vi "my_4th_vi_noloop.vi"(9 "error in (no error)":errorcluster, 10 "Color range":T2, 11 "PNG file":path) -> (2 "error out":errorcluster, 3 "Billard rect":T1)   [LabVIEW 2019]
uses:
  <vilib>/Analysis/Matrix/Numeric/Conversions/Array To Matrix - RA2.vi
  <vilib>/Analysis/Matrix/Numeric/Multiply/Multiply - RM,RM.vi
  <vilib>/Analysis/Matrix/Numeric/Conversions/Matrix To Array - RM.vi
  <vilib>/Analysis/Matrix/Numeric/Conversions/Array To Matrix - RA.vi
  <vilib>/Analysis/Matrix/NI_Matrix.lvlib
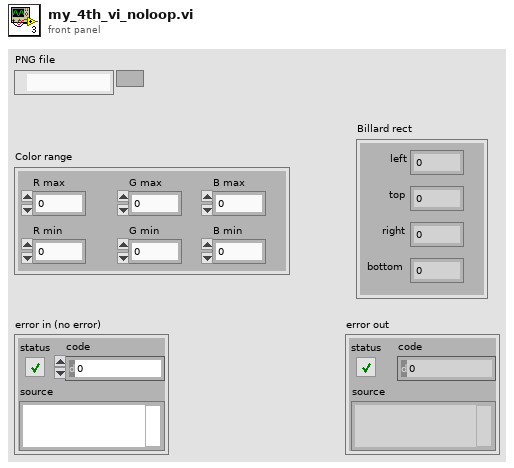
[diagram p1: front panel]
types:
  T1 = cluster{"left":i32, "top":i32, "right":i32, "bottom":i32}
  T2 = cluster{"R max":u8, "R min":u8, "G max":u8, "G min":u8, "B max":u8, "B min":u8}
  T3 = typedef "imagedata.ctl" = cluster{"image type":i32, "image depth":i32, "image":u8[], "mask":u8[], "colors":u32[], "Rectangle":cluster{"left":i16, "top":i16, "right":i16, "bottom":i16}}
  T4 = typedef "NI_Matrix.lvlib/RealMatrix.ctl" = dbl[][]
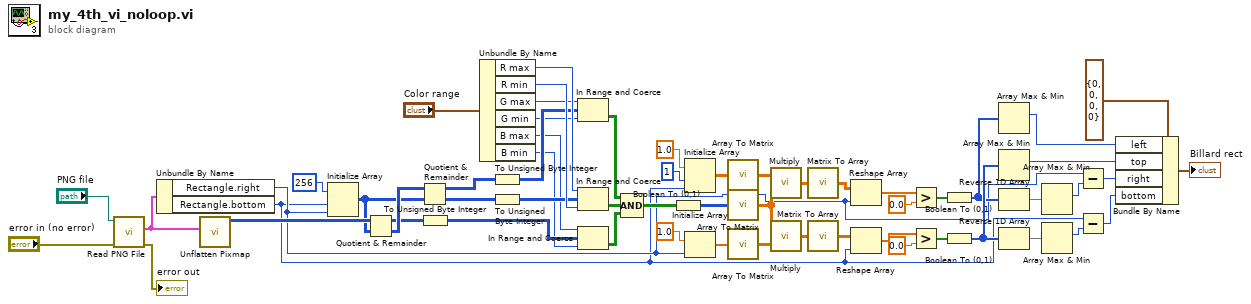
[diagram p0: block diagram]
diagram:
  n1 = call <vilib>:"Read PNG File.vi"("error in (no error)"="error in (no error)", "path to PNG file"="PNG file") -> ("error out"=→"error out":errorcluster, "image data"=w33:T3)  [unwired: 7 in, 1 out]
  n2 = Unbundle By Name(w33) -> ("Rectangle.right"=w4:i16, "Rectangle.bottom"=w2:i16)
  n3 = call <vilib>:"Unflatten Pixmap.vi"("image data"=w33) -> ("24-bit pixmap"=w54:u32[][])  [unwired: 4 in, 6 out]
  n4 = Initialize Array(u32 256 ("element"), w2, w4) -> (w51:u32[][])
  n5 = Quotient & Remainder(x=w54, y=w51) -> (x-y*floor(x/y)=w42:u32[][], floor(x/y)=w52:u32[][])
  n6 = Quotient & Remainder(x=w52, y=w51) -> (x-y*floor(x/y)=w46:u32[][], floor(x/y)=w48:u32[][])
  n7 = To Unsigned Byte Integer(number=w42) -> (unsigned 8bit integer=w41:u8[][])
  n8 = Unbundle By Name("Color range") -> ("R max"=w49:u8, "R min"=w50:u8, "G max"=w44:u8, "G min"=w43:u8, "B max"=w40:u8, "B min"=w39:u8)
  n9 = To Unsigned Byte Integer(number=w46) -> (unsigned 8bit integer=w45:u8[][])
  n10 = To Unsigned Byte Integer(number=w48) -> (unsigned 8bit integer=w47:u8[][])
  n11 = In Range and Coerce(upper limit=w44, x=w45, lower limit=w43) -> (In Range?=w38:bool[][])  [unwired: 1 out]
  n12 = In Range and Coerce(upper limit=w49, x=w47, lower limit=w50) -> (In Range?=w37:bool[][])  [unwired: 1 out]
  n13 = In Range and Coerce(upper limit=w40, x=w41, lower limit=w39) -> (In Range?=w36:bool[][])  [unwired: 1 out]
  n14 = Compound Arithmetic op=AND(w38, w37, w36) -> (w35:bool[][])
  n15 = Boolean To (0,1)(Boolean=w35) -> (0, 1=w34:i16[][])
  n16 = Initialize Array(1.0 ("element"), 1 ("dimension size"), w2) -> (w30:dbl[][])
  n17 = Initialize Array(1.0 ("element"), w4) -> (w31:dbl[])
  n18 = call-poly <vilib>:"Array To Matrix.vi"("Real 2D Array"=w30) -> ("Real Matrix"=w26:T4)
  n19 = call-poly <vilib>:"Array To Matrix.vi"("Real 2D Array"=w34) -> ("Real Matrix"=w25:T4)
  n20 = call-poly <vilib>:"Array To Matrix.vi"("Real 1D Array"=w31) -> ("Real Matrix (Column Vector)"=w29:T4)
  n21 = call-poly <vilib>:"Multiply.vi"("Real Matrix B"=w25, "Real Matrix A"=w26) -> ("A * B"=w24:T4)
  n22 = call-poly <vilib>:"Multiply.vi"("Real Matrix B"=w29, "Real Matrix A"=w25) -> ("A * B"=w23:T4)
  n23 = call-poly <vilib>:"Matrix To Array.vi"("Real Matrix"=w24) -> ("Real 2D Array"=w22:dbl[][])
  n24 = call-poly <vilib>:"Matrix To Array.vi"("Real Matrix"=w23) -> ("Real 2D Array"=w21:dbl[][])
  n25 = Reshape Array(w22, w4) -> (w20:dbl[])
  n26 = Reshape Array(w21, w2) -> (w19:dbl[])
  n27 = Greater?(x=w20, y=0.0) -> (0:w16:bool[])
  n28 = Greater?(x=w19, y=0.0) -> (0:w15:bool[])
  n29 = Boolean To (0,1)(Boolean=w16) -> (0, 1=w12:i16[])
  n30 = Boolean To (0,1)(Boolean=w15) -> (0, 1=w14:i16[])
  n31 = Array Max & Min(array=w12) -> (max index (indices)=w8:i32)  [unwired: 3 out]
  n32 = Array Max & Min(array=w14) -> (max index (indices)=w7:i32)  [unwired: 3 out]
  n33 = Reverse 1D Array(array=w12) -> (reversed array=w11:i16[])
  n34 = Reverse 1D Array(array=w14) -> (reversed array=w13:i16[])
  n35 = Array Max & Min(array=w11) -> (max index (indices)=w3:i32)  [unwired: 3 out]
  n36 = Array Max & Min(array=w13) -> (max index (indices)=w1:i32)  [unwired: 3 out]
  n37 = Subtract(x=w4, y=w3) -> (x-y=w6:i32)
  n38 = Subtract(x=w2, y=w1) -> (x-y=w5:i32)
  n39 = Bundle By Name(cluster=T1 {"left"=0, "top"=0, "right"=0, "bottom"=0} ("Billard rect"), "left"=w8, "top"=w7, "right"=w6, "bottom"=w5) -> (→"Billard rect":T1)
